vi "LI-7000_TH_v01 from Sigi.vi"() -> ()   [LabVIEW 2010]
doc: "This vi is for communication with the infra-red gas analyser LI-7000.\n\nBy Thomas Hombach"
uses:
  <vilib>/Instr/_visa.llb/VISA Configure Serial Port (Instr).vi
panel:
  in  "VISA resource name":refnum<visa-resource-name>="COM11"
  in  "stop":bool
  out "read buffer":string
  out "error out":errorcluster
  out "CO2A":dbl format="%.1f"
  out "CO2B":dbl format="%.1f"
  out "H2OB":dbl format="%.1f"
  out "DH2O (mmol/mol)":dbl format="%.1f"
  out "P (kPa)":dbl format="%.1f"
  out "T (°C)":dbl format="%.1f"
  out "DCO2 (µmol/mol)":dbl format="%.1f"
  out "H2OA":dbl format="%.1f"
  out "LI-COR data":dbl[](array[numeric])
  # "LI-7000"
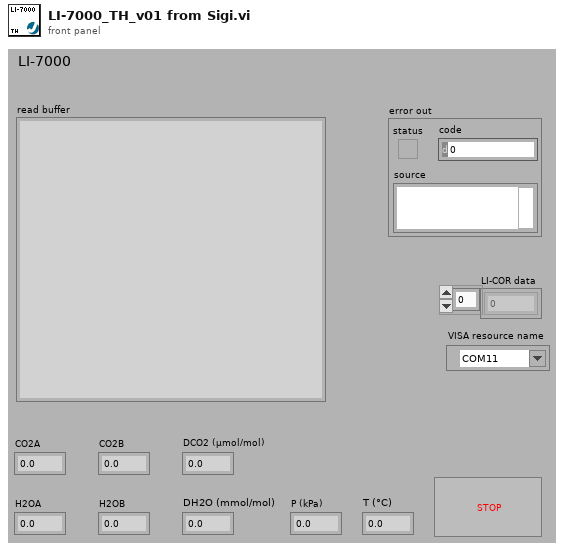
[diagram p1: front panel]
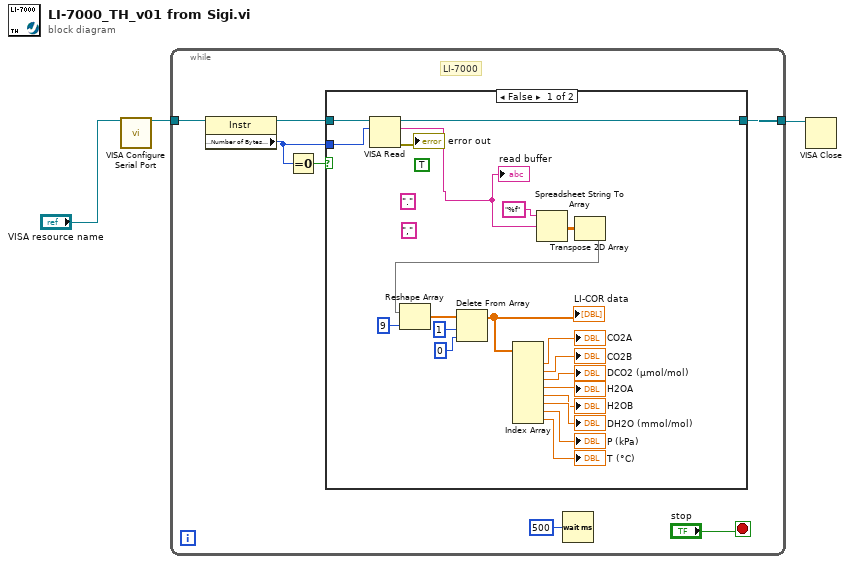
[diagram p0: block diagram]
diagram:
  n1 = call-poly "VISA Configure Serial Port"("VISA resource name"="VISA resource name") -> ("VISA resource name out"=w3:refnum<visa-resource-name>)  [unwired: 5 in, 9 out]
  n2 = while {
    tunnel: w3 -> [w10]
    tunnel: [w6] -> w1
    stop <- "stop" stop-if-true
    # "LI-7000"
    n3 = property class="Instr"(reference=w10) -> (reference out=w8:refnum<visa-resource-name>, "Serial Settings:Number of Bytes at Serial Port"=w7:u32)  [unwired: 1 in, 1 out]
    n4 = Equal To 0?(x=w7) -> (x = 0?=w9:bool)
    n5 = case shown="False" w9 {
      tunnel: w8 -> [w31 w32]
      tunnel: w7 -> [w30 _]
      tunnel: [w29 w32] -> w6
      frame False {
        (unwired) TRUE ("replace all? (F)")
        (unwired) "," ("replace string (\"\")")
        (unwired) "." ("search string")
        n6 = VISA Read(VISA resource name=w31, byte count=w30) -> (VISA resource name out=w29:refnum<visa-resource-name>, read buffer=w11:string, error out=→"error out":errorcluster)  [unwired: 1 in, 1 out]
        "read buffer" <- w11
        n7 = Spreadsheet String To Array(format string="%f", spreadsheet string=w11) -> (array=w27:dbl[][])  [unwired: 2 out]
        n8 = Transpose 2D Array(2D array=w27) -> (transposed array=w26:dbl[][])
        n9 = Reshape Array(w26, 9 ("dimension size")) -> (w24:dbl[])
        n10 = Delete From Array(array=w24, length=1, index=0) -> (array with subset deleted=w20:dbl[])  [unwired: 1 out]
        "LI-COR data" <- w20
        n11 = Index Array(array=w20) -> (element #1=→"CO2A":dbl, element #2=→"CO2B":dbl, element #3=→"DCO2 (µmol/mol)":dbl, element #4=→"H2OA":dbl, element #5=→"H2OB":dbl, element #6=→"DH2O (mmol/mol)":dbl, element #7=→"P (kPa)":dbl, element #8=→"T (°C)":dbl)  [unwired: 8 in]
      }
      frame True {
      }
    }
    n12 = Wait (ms)(milliseconds to wait=u32 500) -> ()  [unwired: 1 out]
  }
  n13 = VISA Close(VISA resource name=w1) -> ()  [unwired: 1 in, 1 out]
